vi "Remote.TCP-IP Listener, Convert JSON to Function Call.vi"(11 "JSON":string="{\n  \"Seq\":0,\n  \"Funct\":\"FunctionName\",\n  \"Args\":\n        [\n        \"Arg1\",\n        \"Arg2\"\n        ]\n}\n") -> (0 "error out":errorcluster, 1 "Args":string[](array[string]), 2 "Function":string, 3 "Seq":i32, 5 "Timeout":dbl)   [LabVIEW 2018]
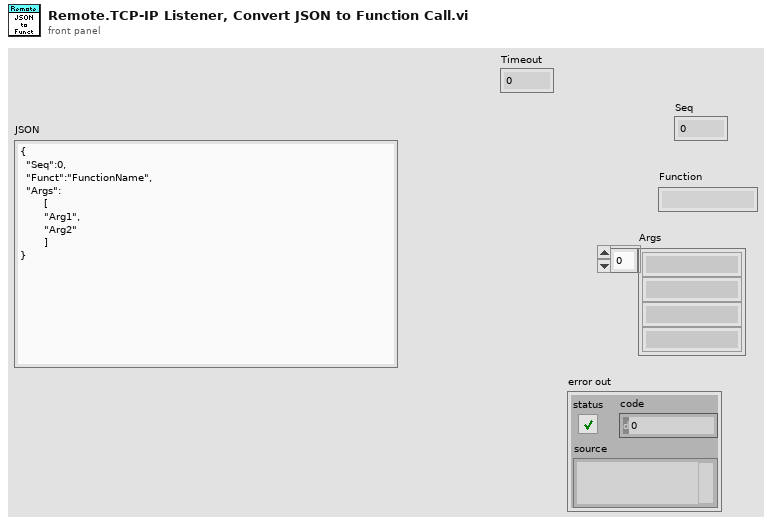
[diagram p1: front panel]
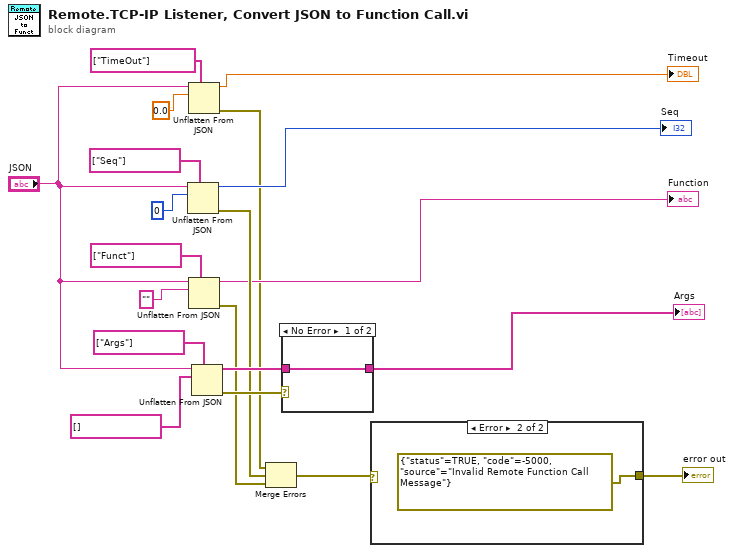
[diagram p0: block diagram]
diagram:
  n1 = Unflatten From JSON(path=string[] ["Seq"], JSON string="JSON", type and defaults=0) -> (value=→"Seq":i32, error out=w9:errorcluster)  [unwired: 4 in]
  n2 = Unflatten From JSON(path=string[] ["TimeOut"], JSON string="JSON", type and defaults=0.0) -> (value=→"Timeout":dbl, error out=w1:errorcluster)  [unwired: 4 in]
  n3 = Unflatten From JSON(path=string[] ["Funct"], JSON string="JSON", type and defaults="") -> (value=→"Function":string, error out=w10:errorcluster)  [unwired: 4 in]
  n4 = Unflatten From JSON(path=string[] ["Args"], JSON string="JSON", type and defaults=string[] []) -> (value=w12:string[], error out=w13:errorcluster)  [unwired: 4 in]
  n5 = Merge Errors(w1, w9, w10) -> (w7:errorcluster)
  n6 = case shown="No Error" w13 {
    tunnel: w12 -> [w21 _]
    tunnel: [w21 _] -> w11
    frame No Error {
    }
    frame Error {
    }
  }
  "Args" <- w11
  n7 = case shown="Error" w7 {
    tunnel: [_ errorcluster {"status"=TRUE, "code"=-5000, "source"="Invalid Remote Function Call Message"} ("error constant")] -> w6
    frame No Error {
    }
    frame Error {
    }
  }
  "error out" <- w6
